vi "speechrecognition.vi"() -> ()   [LabVIEW 2020]
panel:
  in  "stop":bool
  in  "module path":path
  out "String":string
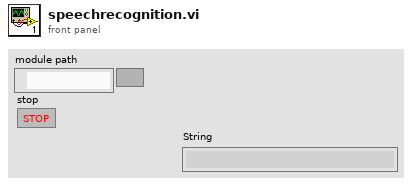
[diagram p1: front panel]
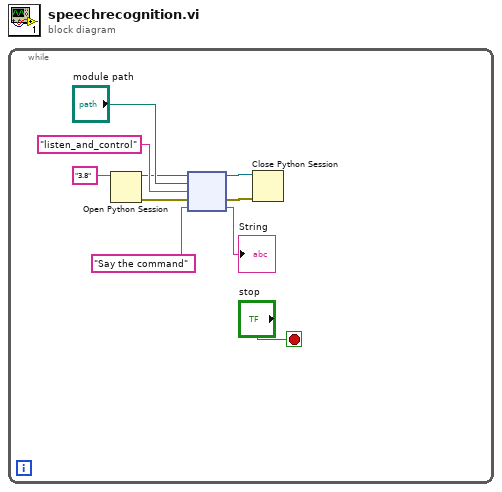
[diagram p0: block diagram]
diagram:
  n1 = while {
    stop <- "stop" stop-if-true
    n2 = Open Python Session(python version="3.8" ("Python version")) -> (session out=w5:refnum<k35>, error out=w4:errorcluster)  [unwired: 2 in]
    n3 = node(w5, "module path", "listen_and_control" ("function name"), w4, "Say the command") -> (w6:refnum<k35>, w3:errorcluster, →"String":string)  [unwired: 2 out]
    n4 = Close Python Session(session in=w6, error in=w3) -> ()  [unwired: 1 out]
  }
